vi "Configure AnalogIn Channel.vi"(0 "ADALM2000 In":u64 caption="Instrument Handle Out", 1 "Trigger enable":bool, 3 "analog_level":dbl, 4 "Range":enum16{"PLUS_MINUS_25_V", "PLUS_MINUS_2_5V"}(ring), 5 "analog_mode":T1, 6 "Channel":T3, 7 "Vertical offset":dbl, 9 "analog_condition":T2) -> (17 "ADALM2000 Out":u64 caption="Instrument Handle Out")   [LabVIEW 2022 SP3]
uses:
  Controls/AnalogChannel.ctl
  Controls/AnalogTriggerCondition.ctl
  Controls/AnalogTriggerMode.ctl
  libm2k_lv.dll
panel:
  in  "Enable":bool
  # "TRIGGER SETTINGS FOR CHANNEL"
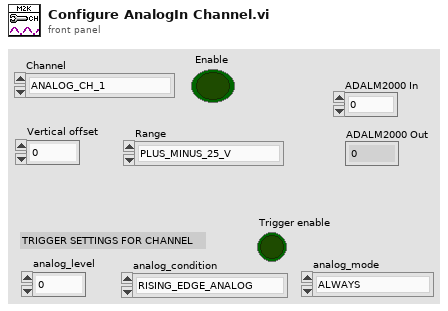
[diagram p1: front panel]
types:
  T1 = typedef "AnalogTriggerMode.ctl" = enum16{"ALWAYS", "ANALOG"}
  T2 = typedef "AnalogTriggerCondition.ctl" = enum16{"RISING_EDGE_ANALOG", "FALLING_EDGE_ANALOG", "LOW_LEVEL_ANALOG", "HIGH_LEVEL_ANALOG"}
  T3 = typedef "AnalogChannel.ctl" = enum16{"ANALOG_CH_1", "ANALOG_CH_2"}
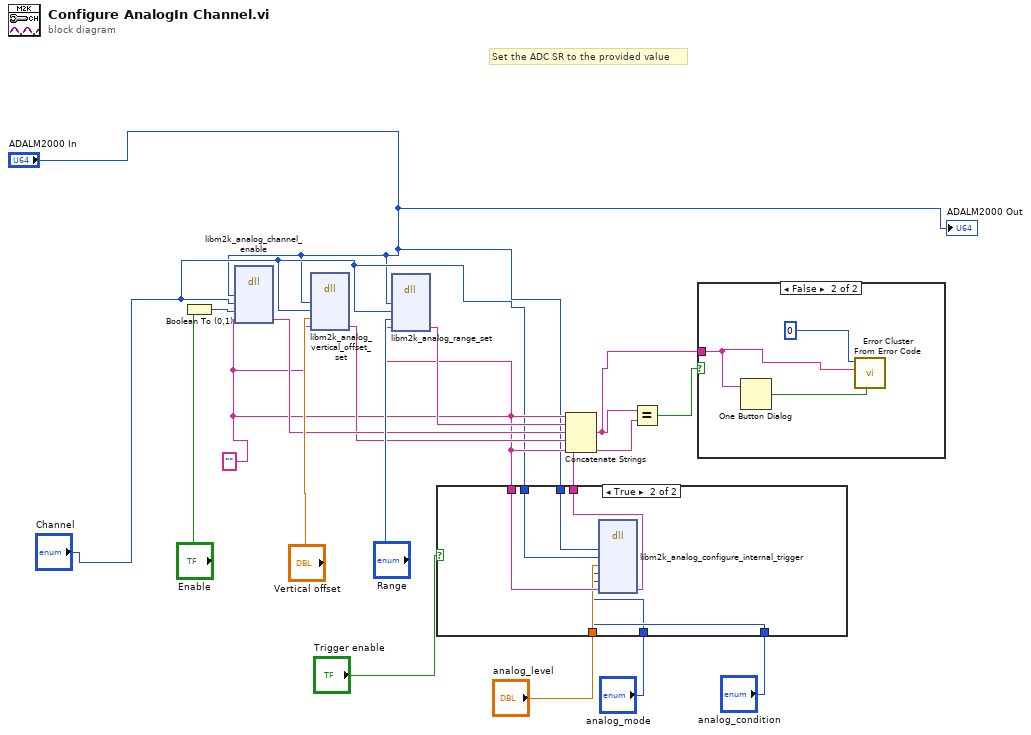
[diagram p0: block diagram]
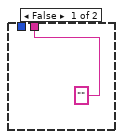
[diagram p2: hidden frame]
diagram:
  w6 = ""
  # "Set the ADC SR to the provided value"
  n1 = Boolean To (0,1)(Boolean="Enable") -> (0, 1=w14:i16)
  n2 = dll-call lib="libm2k_lv.*" fn="libm2k_analog_channel_enable"("instance"="ADALM2000 In", "channel"="Channel", "enable"=w14, "err"=w6) -> ("err"=w13:string)  [unwired: 7 in, 2 out]
  n3 = dll-call lib="libm2k_lv.*" fn="libm2k_analog_vertical_offset_set"("instance"="ADALM2000 In", "channel"="Channel", "vertical_offset"="Vertical offset", "err"=w6) -> ("err"=w12:string)  [unwired: 7 in, 2 out]
  n4 = dll-call lib="libm2k_lv.*" fn="libm2k_analog_range_set"("instance"="ADALM2000 In", "channel"="Channel", "range"="Range", "err"=w6) -> ("err"=w11:string)  [unwired: 7 in, 2 out]
  n5 = case shown="True" "Trigger enable" {
    tunnel: ["" w25] -> w7
    tunnel: w6 -> [_ w24]
    tunnel: "Channel" -> [_ w23]
    tunnel: "ADALM2000 In" -> [_ w22]
    tunnel: "analog_level" -> [_ w21]
    tunnel: "analog_condition" -> [_ w20]
    tunnel: "analog_mode" -> [_ w19]
    frame False {
    }
    frame True {
      n6 = dll-call lib="libm2k_lv.*" fn="libm2k_analog_configure_internal_trigger"("instance"=w22, "chnIdx"=w23, "analog_level"=w21, "analog_condition"=w20, "analog_mode"=w19, "err"=w24) -> ("err"=w25:string)  [unwired: 9 in, 2 out]
    }
  }
  n7 = Concatenate Strings(w6, w11, w13, w12, w7) -> (w9:string)
  n8 = Equal?(x=w9, y=w6) -> (x = y?=w10:bool)
  n9 = case shown="False" w10 {
    tunnel: w9 -> [_ w26]
    frame True {
    }
    frame False {
      n10 = One Button Dialog(message=w26) -> (true=w28:bool)  [unwired: 1 in]
      n11 = call <vilib>:"Error Cluster From Error Code.vi"("show call chain? (False)"=w28, "error message (\"\")"=w26, "error code (0)"=0) -> ()  [unwired: 6 in, 1 out]
    }
  }
  "ADALM2000 Out" <- "ADALM2000 In"
